vi "Read & Decode PTU Data v4.vi"(0 "Byte Stream File in":refnum<file>, 5 "PicoQuant Data File Information":T1, 9 "Multiframe Readout":bool, 11 "error in (no error)":errorcluster) -> (1 "Frame Timestamps (s)":dbl[](array[numeric]), 2 "Frame Start Indices":i32[](array[numeric]), 3 "Time (s)":dbl, 4 "Macrotimes":u64[](array[numeric]), 6 "Nanotimes":u32[](array[numeric]), 8 "Channels":u8[](array[numeric]), 10 "# Frames (inferred)":i32, 13 "Pixel Durations (inferred_":i64[](array[numeric]), 14 "Line Start Macrotimes":u64[](array[numeric]), 15 "Error Out":errorcluster)   [LabVIEW 2021, in "PTU Files.lvlib"]
uses:
  PTU Files.lvlib
  PicoQuant Data File Information.ctl
  PicoQuant File Information.ctl
  PicoQuant Software Information.ctl
  PicoQuant Remote Request Information.ctl
  PicoQuant Hardware Information.ctl
  PicoQuant Input Channels.ctl
  PicoQuant Markers.ctl
  PicoQuant Modules.ctl
  PicoQuant Router Channels.ctl
  PicoQuant Measurement Information.ctl
  PicoQuant Image Information.ctl
  PicoQuant Results Format.ctl
  PicoQuant Measurement Results.ctl
  0aca7642-3e1d-4496-a7c2-816a246d9d6f.vi
  b41b1344-b631-4a7f-8889-5162ffc345c0.vi
  Time/Time.lvlib
  Utilities/Utilities.lvlib
panel:
  out "Pixel Durations":i64[](array[numeric])
  out "Frame Marker Macrotimes":u64[](array[numeric])
  out "Line Stop Macrotimes":u64[](array[numeric])
  out "# Frame Markers":i32
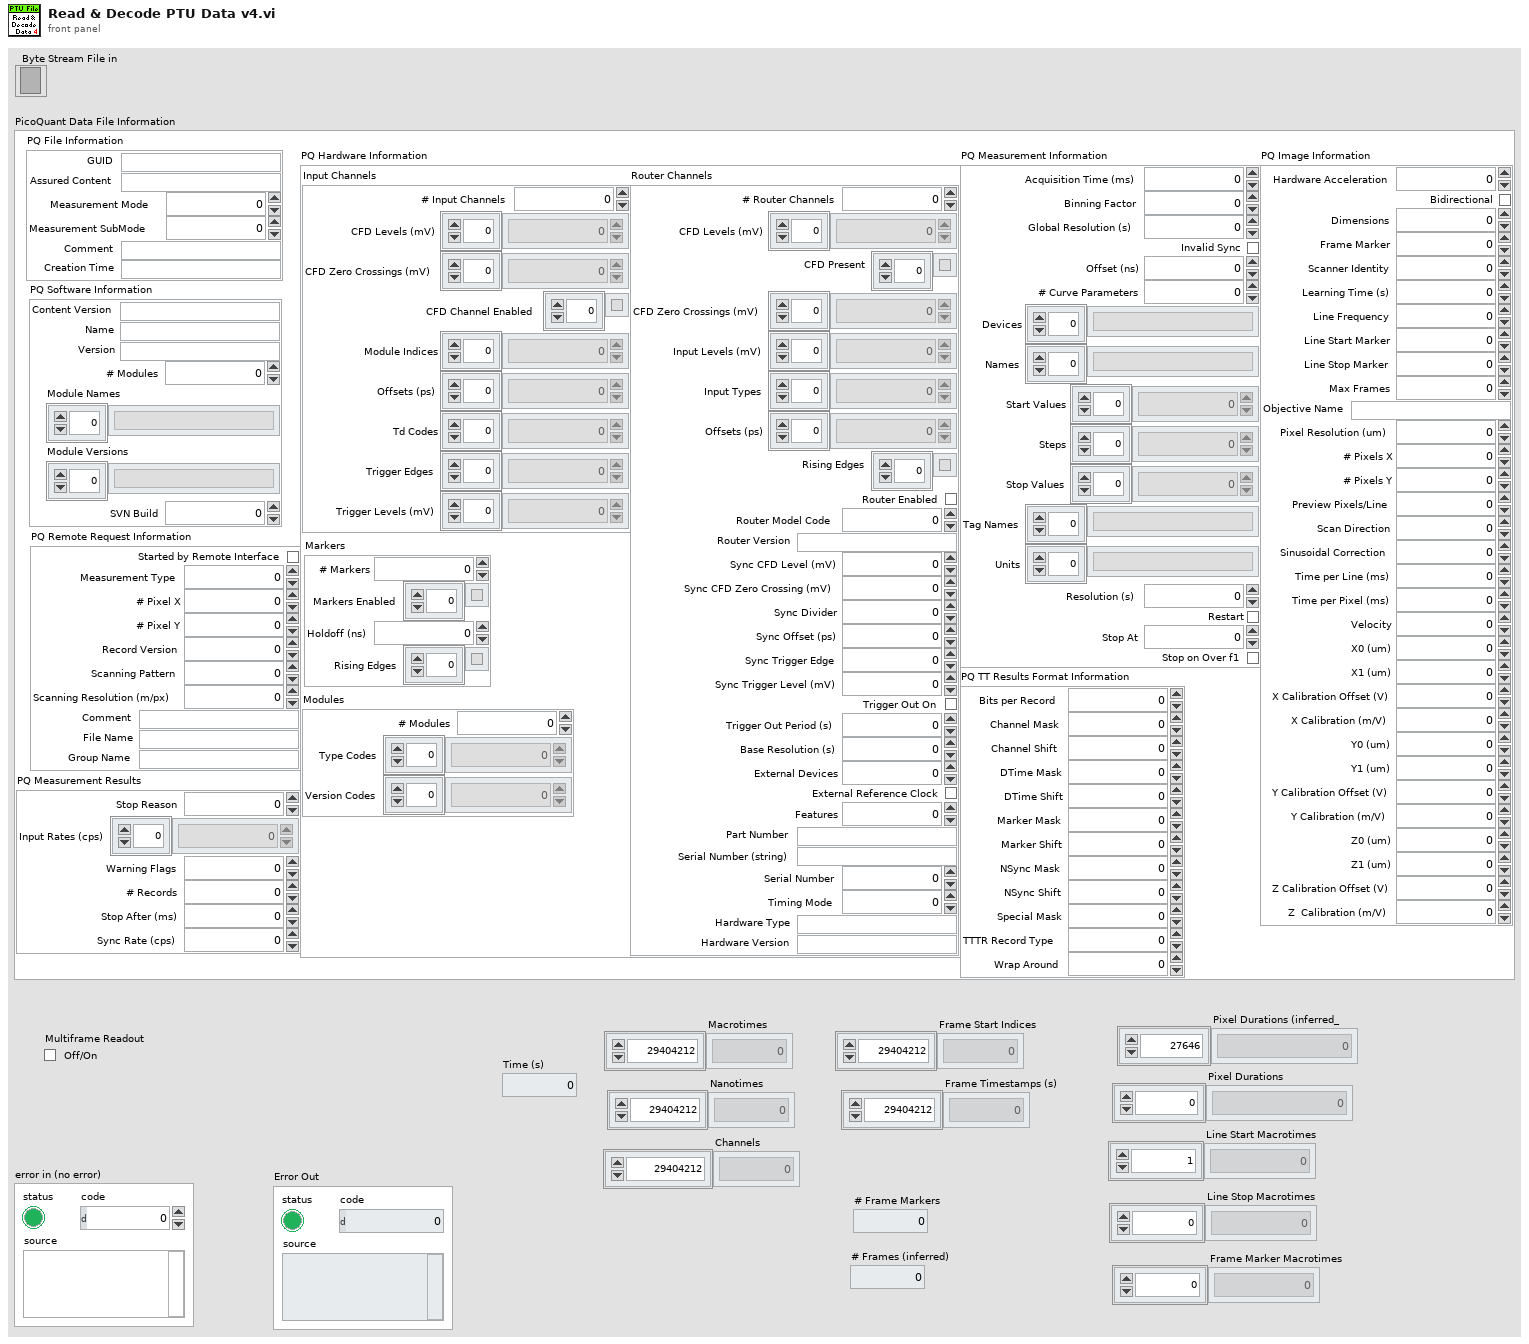
[diagram p1: front panel]
types:
  T1 = typedef "PTU Files.lvlib/PicoQuant Data File Information.ctl" = cluster{"PQ File Information":T2, "PQ Software Information":T3, "PQ Remote Request Information":T4, "PQ Hardware Information":T5, "PQ Measurement Information":T10, "PQ Image Information":T11, "PQ TT Results Format Information":T12, "PQ Measurement Results":T13}
  T2 = typedef "PTU Files.lvlib/PicoQuant File Information.ctl" = cluster{"GUID":string, "Assured Content":string, "Measurement Mode":i64, "Measurement SubMode":i64, "Comment":string, "Creation Time":string}
  T3 = typedef "PTU Files.lvlib/PicoQuant Software Information.ctl" = cluster{"Content Version":string, "Name":string, "Version":string, "# Modules":i64, "Module Names":string[], "Module Versions":string[], "SVN Build":i64}
  T4 = typedef "PTU Files.lvlib/PicoQuant Remote Request Information.ctl" = cluster{"Started by Remote Interface":bool, "Measurement Type":i64, "# Pixel X":i64, "# Pixel Y":i64, "Record Version":i64, "Scanning Pattern":i64, "Scanning Resolution (m/px)":dbl, "Comment":string, "File Name":string, "Group Name":string}
  T5 = typedef "PTU Files.lvlib/PicoQuant Hardware Information.ctl" = cluster{"Input Channels":T6, "Markers":T7, "Modules":T8, "Router Channels":T9}
  T6 = typedef "PTU Files.lvlib/PicoQuant Input Channels.ctl" = cluster{"# Input Channels":i64, "CFD Levels (mV)":i64[], "CFD Zero Crossings (mV)":i64[], "CFD Channel Enabled":bool[], "Module Indices":i64[], "Offsets (ps)":i64[], "Td Codes":i64[], "Trigger Edges":i64[], "Trigger Levels (mV)":i64[]}
  T7 = typedef "PTU Files.lvlib/PicoQuant Markers.ctl" = cluster{"# Markers":i64, "Markers Enabled":bool[], "Holdoff (ns)":i64, "Rising Edges":bool[]}
  T8 = typedef "PTU Files.lvlib/PicoQuant Modules.ctl" = cluster{"# Modules":i64, "Type Codes":i64[], "Version Codes":i64[]}
  T9 = typedef "PTU Files.lvlib/PicoQuant Router Channels.ctl" = cluster{"# Router Channels":i64, "CFD Levels (mV)":i64[], "CFD Present":bool[], "CFD Zero Crossings (mV)":i64[], "Input Levels (mV)":i64[], "Input Types":i64[], "Offsets (ps)":i64[], "Rising Edges":bool[], "Router Enabled":bool, "Router Model Code":i64, "Router Version":string, "Sync CFD Level (mV)":i64, "Sync CFD Zero Crossing (mV)":i64, "Sync Divider":i64, "Sync Offset (ps)":i64, "Sync Trigger Edge":i64, "Sync Trigger Level (mV)":i64, "Trigger Out On":bool, "Trigger Out Period (s)":dbl, "Base Resolution (s)":dbl, "External Devices":i64, "External Reference Clock":bool, "Features":u64, "Part Number":string, "Serial Number (string)":string, "Serial Number":i64, "Timing Mode":i64, "Hardware Type":string, "Hardware Version":string}
  T10 = typedef "PTU Files.lvlib/PicoQuant Measurement Information.ctl" = cluster{"Acquisition Time (ms)":i64, "Binning Factor":i64, "Global Resolution (s)":dbl, "Invalid Sync":bool, "Offset (ns)":u64, "# Curve Parameters":u64, "Devices":string[], "Names":string[], "Start Values":dbl[], "Steps":dbl[], "Stop Values":dbl[], "Tag Names":string[], "Units":string[], "Resolution (s)":dbl, "Restart":bool, "Stop At":u64, "Stop on Over f1":bool}
  T11 = typedef "PTU Files.lvlib/PicoQuant Image Information.ctl" = cluster{"Hardware Acceleration":i64, "Bidirectional":bool, "Dimensions":i64, "Frame Marker":i64, "Scanner Identity":i64, "Learning Time (s)":i64, "Line Frequency":dbl, "Line Start Marker":i64, "Line Stop Marker":i64, "Max Frames":i64, "Objective Name":string, "Pixel Resolution (um)":dbl, "# Pixels X":i64, "# Pixels Y":i64, "Preview Pixels/Line":i64, "Scan Direction":i64, "Sinusoidal Correction":i64, "Time per Line (ms)":dbl, "Time per Pixel (ms)":i64, "Velocity":i64, "X0 (um)":dbl, "X1 (um)":dbl, "X Calibration Offset (V)":dbl, "X Calibration (m/V)":dbl, "Y0 (um)":dbl, "Y1 (um)":dbl, "Y Calibration Offset (V)":dbl, "Y Calibration (m/V)":dbl, "Z0 (um)":dbl, "Z1 (um)":dbl, "Z Calibration Offset (V)":dbl, "Z  Calibration (m/V)":dbl}
  T12 = typedef "PTU Files.lvlib/PicoQuant Results Format.ctl" = cluster{"Bits per Record":i64, "Channel Mask":i64, "Channel Shift ":i64, "DTime Mask":i64, "DTime Shift":i64, "Marker Mask":i64, "Marker Shift":i64, "NSync Mask":i64, "NSync Shift":i64, "Special Mask":i64, "TTTR Record Type":i64, "Wrap Around":i64}
  T13 = typedef "PTU Files.lvlib/PicoQuant Measurement Results.ctl" = cluster{"Stop Reason":i64, "Input Rates (cps)":i64[], "Warning Flags":u64, "# Records":i64, "Stop After (ms)":i64, "Sync Rate (cps)":i64}
  T14 = enum16{"big-endian, network order", "native, host order", "little-endian"}
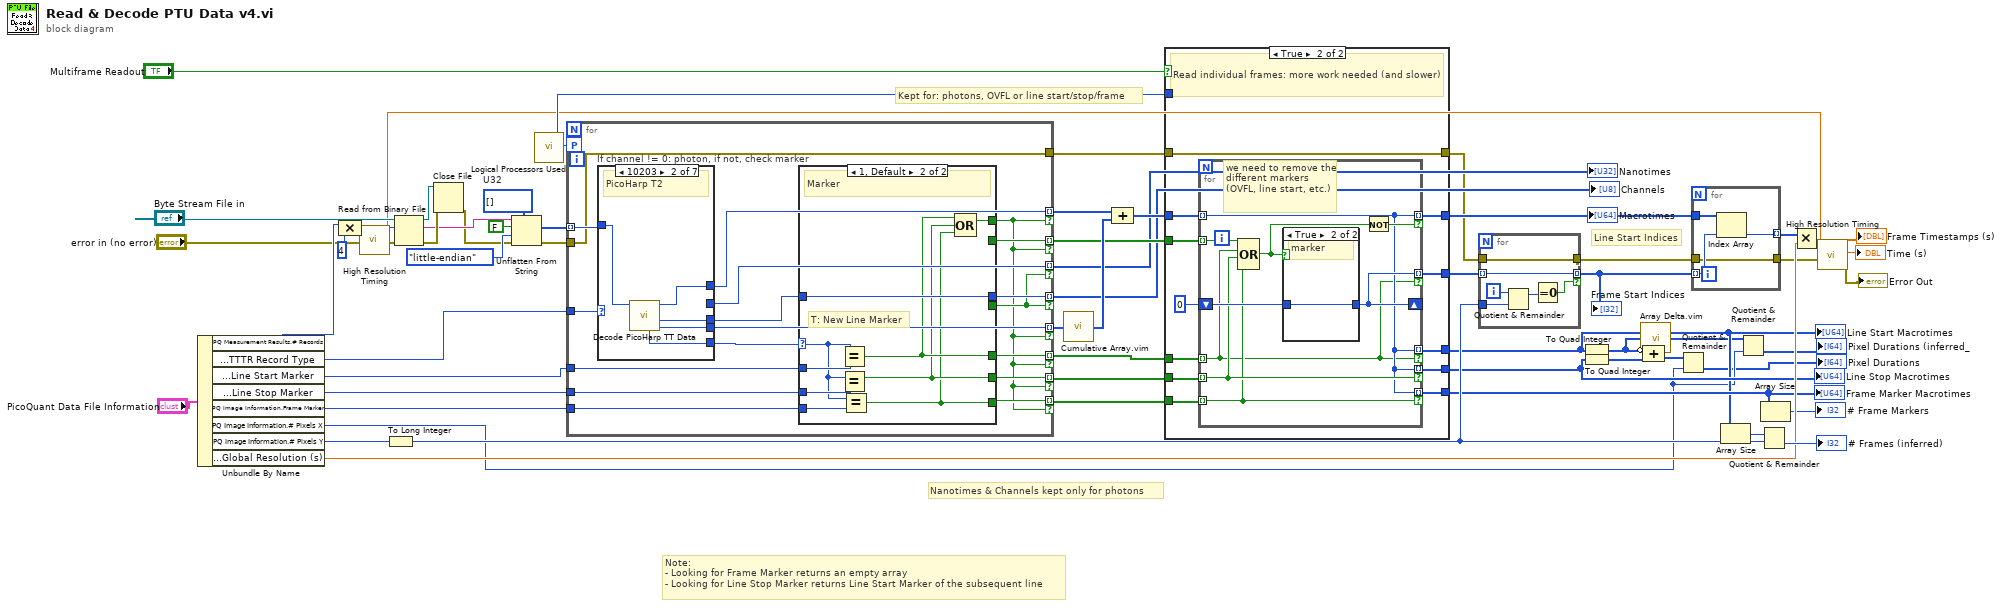
[diagram p0: block diagram]
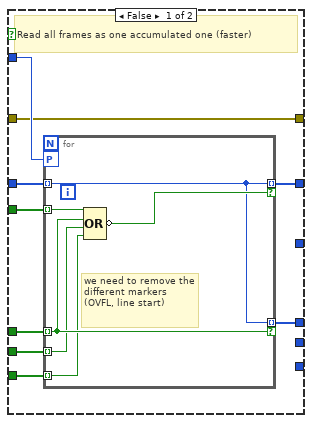
[diagram p2: hidden frame]
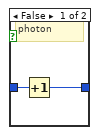
[diagram p3: hidden frame]
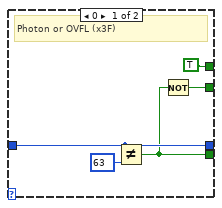
[diagram p4: hidden frame]
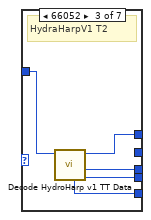
[diagram p6: hidden frame]
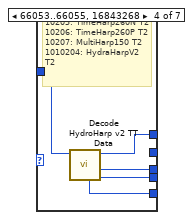
[diagram p7: hidden frame]
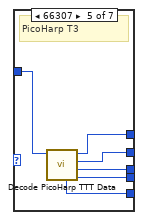
[diagram p8: hidden frame]
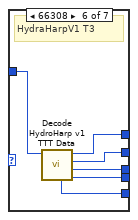
[diagram p9: hidden frame]
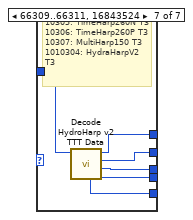
[diagram p10: hidden frame]
diagram:
  w50 = u32[] []  # U32
  # "Note:\n- Looking for Frame Marker returns an empty array\n- Looking for Line Stop Marker returns Line Start Marker of the subsequent line"
  # "Line Start Indices"
  # "Kept for: photons, OVFL or line start/stop/frame"
  # "Nanotimes & Channels kept only for photons"
  n1 = Unbundle By Name("PicoQuant Data File Information") -> ("PQ Measurement Results.# Records"=w58:i64, "PQ TT Results Format Information.TTTR Record Type"=w57:i64, "PQ Image Information.Line Start Marker"=w56:i64, "PQ Image Information.Line Stop Marker"=w18:i64, "PQ Image Information.Frame Marker"=w17:i64, "PQ Image Information.# Pixels X"=w3:i64, "PQ Image Information.# Pixels Y"=w37:i64, "PQ Measurement Information.Global Resolution (s)"=w26:dbl)
  n2 = Compound Arithmetic op=MULTIPLY(w58, i64 4) -> (w54:i64)
  n3 = call "High Resolution Timing.vi"("Error In"="error in (no error)") -> ("elapsed (relative) seconds"=w22:dbl, "Error Out"=w45:errorcluster)  [unwired: 16 in, 1 out]
  n4 = To Long Integer(number=w37) -> (32bit integer=w16:i32)
  n5 = Read from Binary File(8:w45, 10:w54, 11:"Byte Stream File in") -> (0:w52:errorcluster, 2:w51:string, 3:w53:refnum<file>)  [unwired: 3 in, 1 out]
  n6 = Close File(refnum=w53, error in=w52) -> (error out=w44:errorcluster)  [unwired: 1 out]
  n7 = Unflatten From String(type=w50, binary string=w51, data includes array or string size? (T)=FALSE, byte order (0:big-endian, network order)=T14."little-endian", error in (no error)=w44) -> (value=w47:u32[], error out=w43:errorcluster)  [unwired: 1 out]
  n8 = call "Logical Processors Used.vi"() -> ("# Logical Processor Used"=w29:i32)  [unwired: 6 in]
  n9 = for {
    tunnel: w57 -> [w78]
    tunnel: w56 -> [w75]
    tunnel: w47 -> [w74] mode=indexing
    tunnel: [w73] -> w33 mode=indexing if=w67
    tunnel: [w72] -> w36 mode=indexing if=w61
    tunnel: [w71] -> w32 mode=indexing if=w67
    tunnel: w43 -> [w70]
    tunnel: [w70] -> w21
    tunnel: [w69] -> w40 mode=indexing if=w61
    tunnel: [w68] -> w38 mode=indexing if=w61
    tunnel: [w66] -> w34 mode=indexing if=w61
    workers-P: w29 -> [_]
    tunnel: w18 -> [w65]
    tunnel: w17 -> [w64]
    tunnel: [w63] -> w15 mode=indexing if=w61
    tunnel: [w62] -> w14 mode=indexing if=w61
    n10 = case "If channel != 0: photon, if not, check marker" shown="10203" w78 {
      tunnel: [_ w95 w99 w106 w110 w117 w121] -> w69
      tunnel: [_ w94 w98 w103 w109 w118 w120] -> w77
      tunnel: [_ w96 w101 w105 w113 w116 w124] -> w72
      tunnel: [_ _ _ _ w112 w115 w123] -> w73
      tunnel: [_ w93 w100 w104 w111 w114 w122] -> w76
      tunnel: w74 -> [_ w97 w102 w107 w108 w119 w125]
      frame Default {
        # "unknown record type"
      }
      frame 66051 {
        # "PicoHarp T2"
        n11 = call "Decode PicoHarp TT Data.vi"("rawbits"=w97) -> ("oflcorr_out"=w95:u64, "channel"=w93:u8, "truetime"=w96:u64, "markercode"=w94:u32)  [unwired: 7 in]
      }
      frame 66052 {
        # "HydraHarpV1 T2"
        n12 = call "Decode HydroHarp v1 TT Data.vi"("rawbits"=w102) -> ("oflcorr_out"=w99:u64, "channel"=w100:u8, "truetime"=w101:u64, "markercode"=w98:u32)  [unwired: 7 in]
      }
      frame 66053..66055, 16843268 {
        # "10205: TimeHarp260N T2\n10206: TimeHarp260P T2 \n10207: MultiHarp150 T2\n1010204: HydraHarpV2 T2"
        n13 = call "Decode HydroHarp v2 TT Data.vi"("rawbits"=w107) -> ("oflcorr_out"=w106:u64, "channel"=w104:u8, "truetime"=w105:u64, "markercode"=w103:u32)  [unwired: 7 in]
      }
      frame 66307 {
        # "PicoHarp T3"
        n14 = call "Decode PicoHarp TTT Data.vi"("rawbits"=w108) -> ("oflcorr_out"=w110:u64, "channel"=w111:u8, "dtime"=w112:u32, "truetime"=w113:u64, "markercode"=w109:u32)  [unwired: 6 in]
      }
      frame 66308 {
        # "HydraHarpV1 T3"
        n15 = call "Decode HydroHarp v1 TTT Data.vi"("rawbits"=w119) -> ("oflcorr_out"=w117:u64, "channel"=w114:u8, "dtime"=w115:u32, "truetime"=w116:u64, "markercode"=w118:u32)  [unwired: 6 in]
      }
      frame 66309..66311, 16843524 {
        # "10305: TimeHarp260N T3\n10306: TimeHarp260P T3\n10307: MultiHarp150 T3\n1010304: HydraHarpV2 T3"
        n16 = call "Decode HydroHarp v2 TTT Data.vi"("rawbits"=w125) -> ("oflcorr_out"=w121:u64, "channel"=w122:u8, "dtime"=w123:u32, "truetime"=w124:u64, "markercode"=w120:u32)  [unwired: 6 in]
      }
    }
    n17 = case shown="1, Default" w77 {
      selector: w77 -> [_ w87]
      tunnel: w76 -> [w83 w91]
      tunnel: w75 -> [_ w92]
      tunnel: [TRUE w86] -> w61
      tunnel: [w83 w91] -> w71
      tunnel: [_ w90] -> w68
      tunnel: [w80 _] -> w67
      tunnel: [w79 _] -> w66
      tunnel: w65 -> [_ w89]
      tunnel: w64 -> [_ w88]
      tunnel: [_ w84] -> w63
      tunnel: [_ w85] -> w62
      frame 0 {
        # "Photon or OVFL (x3F)"
        n18 = Not Equal?(x=w83, y=u8 63) -> (x != y?=w80:bool)
        n19 = Not(x=w80) -> (.not. x?=w79:bool)
      }
      frame 1, Default {
        # "T: New Line Marker"
        # "Marker"
        n20 = Equal?(x=w87, y=w92) -> (x = y?=w90:bool)
        n21 = Equal?(x=w87, y=w89) -> (x = y?=w85:bool)
        n22 = Equal?(x=w87, y=w88) -> (x = y?=w84:bool)
        n23 = Compound Arithmetic op=OR(w90, w85, w84) -> (w86:bool)
      }
    }
  }
  "Nanotimes" <- w33
  "Channels" <- w32
  n24 = call "Cumulative Array.vim"("Array"=w40) -> ("cumulative Array"=w35:u64[])  [unwired: 8 in]
  n25 = Compound Arithmetic op=ADD(w36, w35) -> (w39:u64[])
  n26 = case shown="True" "Multiframe Readout" {
    tunnel: w39 -> [w134 w152]
    tunnel: w38 -> [w133 w151]
    tunnel: [w132 w150] -> w28
    tunnel: [w131 w149] -> w6
    tunnel: w34 -> [w130 w148]
    tunnel: [_ w146] -> w31
    tunnel: w29 -> [w129 _]
    tunnel: w21 -> [w128 w145]
    tunnel: [w128 w145] -> w25
    tunnel: w15 -> [w127 w144]
    tunnel: w14 -> [w126 w143]
    tunnel: [_ w142] -> w10
    tunnel: [_ w141] -> w9
    frame False {
      # "Read all frames as one accumulated one (faster)"
      n27 = for {
        tunnel: w134 -> [w137] mode=indexing
        tunnel: w133 -> [w138] mode=indexing
        tunnel: [w137] -> w132 mode=indexing if=w139
        tunnel: [w137] -> w131 mode=indexing if=w138
        tunnel: w130 -> [w140] mode=indexing
        workers-P: w129 -> [_]
        tunnel: w127 -> [w136] mode=indexing
        tunnel: w126 -> [w135] mode=indexing
        # "we need to remove the different markers (OVFL, line start)"
        n28 = Compound Arithmetic op=OR(w140, w138, w135, w136) -> (invert w139:bool)
      }
    }
    frame True {
      # "Read individual frames: more work needed (and slower)"
      n29 = for {
        tunnel: w152 -> [w155] mode=indexing
        tunnel: w151 -> [w153] mode=indexing
        tunnel: [w155] -> w150 mode=indexing if=w157
        tunnel: [w155] -> w149 mode=indexing if=w153
        tunnel: w148 -> [w161] mode=indexing
        shift-right: [w158] -> _
        shift-left: 0 -> [w159]
        tunnel: [w158] -> w146 mode=indexing if=w153
        tunnel: w144 -> [w154] mode=indexing
        tunnel: w143 -> [w156] mode=indexing
        tunnel: [w155] -> w142 mode=indexing if=w156
        tunnel: [w155] -> w141 mode=indexing if=w154
        # "we need to remove the different markers (OVFL, line start, etc.)"
        n30 = Compound Arithmetic op=OR(w161, w153, w156, w154) -> (w160:bool)
        n31 = case shown="True" w160 {
          tunnel: w159 -> [w163 w164]
          tunnel: [w162 w164] -> w158
          frame False {
            # "photon"
            n32 = Increment(x=w163) -> (x+1=w162:i32)
          }
          frame True {
            # "marker"
          }
        }
        n33 = Not(x=w160) -> (.not. x?=w157:bool)
      }
    }
  }
  "Line Start Macrotimes" <- w6
  "Macrotimes" <- w28
  "Line Stop Macrotimes" <- w10
  "Frame Marker Macrotimes" <- w9
  n34 = for {
    tunnel: w31 -> [w168] mode=indexing
    tunnel: w16 -> [w170]
    tunnel: [w168] -> w8 mode=indexing if=w167
    tunnel: [w165] -> w24
    tunnel: w25 -> [w165]
    i -> [w166]
    n35 = Quotient & Remainder(x=w166, y=w170) -> (x-y*floor(x/y)=w169:i32)  [unwired: 1 out]
    n36 = Equal To 0?(x=w169) -> (x = 0?=w167:bool)
  }
  "Frame Start Indices" <- w8
  n37 = To Quad Integer(1:w6) -> (0:w5:i64[])
  n38 = To Quad Integer(1:w10) -> (0:w13:i64[])
  n39 = call "Array Delta.vim"("A"=w5) -> ("A[i+1]-A[i]"=w4:i64[])  [unwired: 8 in]
  n40 = Compound Arithmetic op=ADD(invert w5, w13) -> (w12:i64[])
  n41 = Quotient & Remainder(x=w12, y=w3) -> (floor(x/y)=→"Pixel Durations":i64[])  [unwired: 1 out]
  n42 = for {
    tunnel: w28 -> [w174]
    tunnel: w8 -> [w173] mode=indexing
    tunnel: [w172] -> w27 mode=indexing
    tunnel: w24 -> [w171]
    tunnel: [w171] -> w23
    n43 = Index Array(array=w174, index=w173) -> (element=w172:u64)
  }
  n44 = Array Size(array=w6) -> (size(s)=w42:i32)
  n45 = Quotient & Remainder(x=w4, y=w3) -> (floor(x/y)=→"Pixel Durations (inferred_":i64[])  [unwired: 1 out]
  n46 = Quotient & Remainder(x=w42, y=w16) -> (floor(x/y)=→"# Frames (inferred)":i32)  [unwired: 1 out]
  n47 = Array Size(array=w9) -> (size(s)=→"# Frame Markers":i32)
  n48 = Multiply(x=w27, y=w26) -> (x*y=→"Frame Timestamps (s)":dbl[])
  n49 = call "High Resolution Timing.vi"("relative seconds (NaN)"=w22, "Error In"=w23) -> ("elapsed (relative) seconds"=→"Time (s)":dbl, "Error Out"=→"Error Out":errorcluster)  [unwired: 15 in, 1 out]
